vi "Get Common Elements from 2 Arrays.vi"(0 "Array 1":i32[](array[numeric]), 1 "Array 2":i32[](array[numeric])) -> (12 "Empty?":bool, 14 "Intended Array":i32[](array[numeric]), 15 "Common Array":i32[](array[numeric]))   [LabVIEW 2014, in "Dragon Tamers.lvlib"]
uses:
  Dragon Tamers.lvlib
  <userlib>/_OpenG.lib/array/array.llb/Filter 1D Array (I32)__ogtk.vi
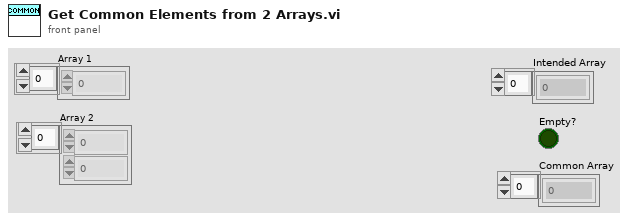
[diagram p1: front panel]
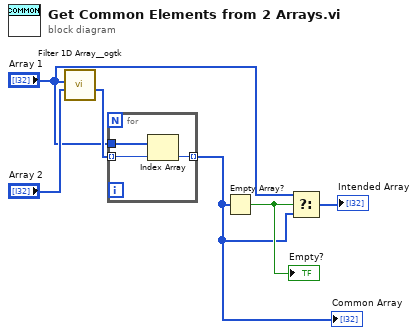
[diagram p0: block diagram]
diagram:
  n1 = call-poly <userlib>:"Filter 1D Array__ogtk.vi"("items to filter"="Array 2", "array"="Array 1") -> ("filtered item indices"=w5:i32[])  [unwired: 4 in, 1 out]
  n2 = for {
    tunnel: w5 -> [w8] mode=indexing
    tunnel: "Array 1" -> [w9]
    tunnel: [w7] -> w3 mode=indexing
    n3 = Index Array(array=w9, index=w8) -> (element=w7:i32)
  }
  "Common Array" <- w3
  n4 = Empty Array?(array=w3) -> (empty?=w4:bool)
  "Empty?" <- w4
  n5 = Select(t="Array 1", s=w4, f=w3) -> (s? t:f=→"Intended Array":i32[])
